vi "Set_Vsg2.vi"(7 "Numeric":dbl) -> (3 "Numeric 2":dbl)   [LabVIEW 2013]
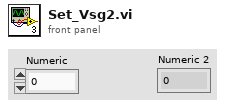
[diagram p1: front panel]
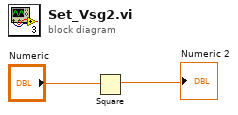
[diagram p0: block diagram]
diagram:
  n1 = Square(x="Numeric") -> (x^2=→"Numeric 2":dbl)
